vi "Create Trigger Model On Event Branch.vi"(0 "VISA resource name":refnum<visa-resource-name>, 5 "Block Number (1)":i32=1 min=1 format="%#.6g", 7 "Stimulus Event":u16(ring) items=["None", "Front Pannel Trigger Key", "Notify Trigger Block 1", "Notify Trigger Block 2", "Notify Trigger Block 3", "Notify Trigger Block 4", "Notify Trigger Block 5", "Notify Trigger Block 6", "Notify Trigger Block 7", "Notify Trigger Block 8", "Command", "Digi IO Line 1", "Digi IO Line 2", "Digi IO Line 3", "Digi IO Line 4", "Digi IO Line 5", "Digi IO Line 6", "TSP-Link 1", "TSP-Link 2", "TSP-Link 3", "LAN 1", "LAN 2", "LAN 3", "LAN 4", "LAN 5", "LAN 6", "LAN 7", "LAN 8", "Blender 1", "Blender 2", "Timer 1", "Timer 2", "Timer 3", "Timer 4", "Analog Trigger", "External Trigger"], 9 "Branch To Block":i32=1 min=1 format="%#.6g", 11 "error in (no error)":errorcluster) -> (4 "VISA resource name out":refnum<visa-resource-name>, 15 "error Out (no error)":errorcluster)   [LabVIEW 2021, in "Keithley DMM7510.lvlib"]
doc: "This VI branches to a specified block when a specified trigger event occurs."
uses:
  Keithley DMM7510.lvlib
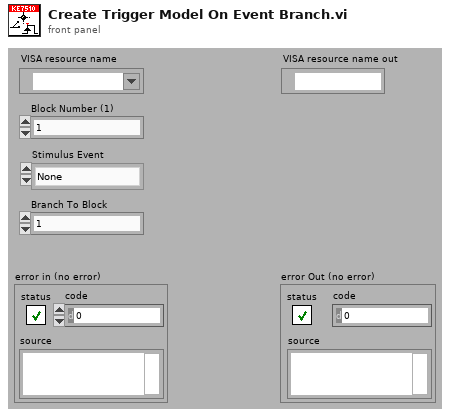
[diagram p1: front panel]
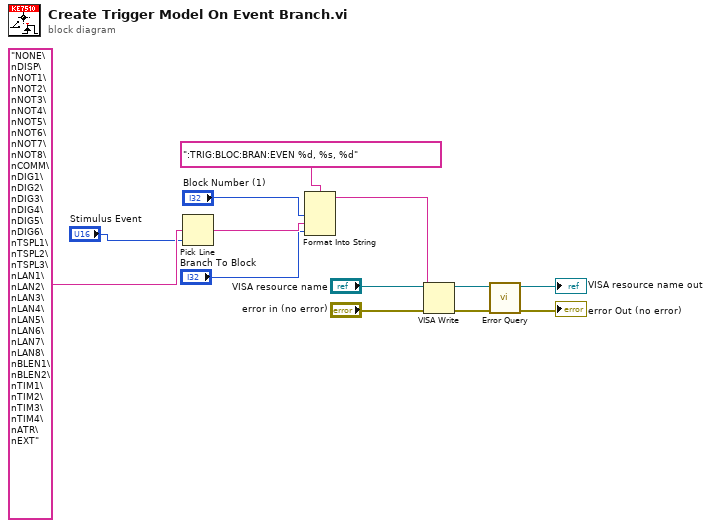
[diagram p0: block diagram]
diagram:
  n1 = Pick Line(multi-line string="NONE\nDISP\nNOT1\nNOT2\nNOT3\nNOT4\nNOT5\nNOT6\nNOT7\nNOT8\nCOMM\nDIG1\nDIG2\nDIG3\nDIG4\nDIG5\nDIG6\nTSPL1\nTSPL2\nTSPL3\nLAN1\nLAN2\nLAN3\nLAN4\nLAN5\nLAN6\nLAN7\nLAN8\nBLEN1\nBLEN2\nTIM1\nTIM2\nTIM3\nTIM4\nATR\nEXT", line index="Stimulus Event") -> (output string=w5:string)  [unwired: 1 in]
  n2 = Format Into String(format string=":TRIG:BLOC:BRAN:EVEN %d, %s, %d", "Block Number (1)", w5, "Branch To Block") -> (resulting string=w11:string)  [unwired: 2 in, 1 out]
  n3 = VISA Write(VISA resource name="VISA resource name", write buffer=w11, error in (no error)="error in (no error)") -> (VISA resource name out=w10:refnum<visa-resource-name>, error out=w9:errorcluster)  [unwired: 1 out]
  n4 = call "Error Query.vi"("error in (no error)"=w9, "VISA resource name"=w10) -> ("error out"=→"error Out (no error)":errorcluster, "VISA resource name out"=→"VISA resource name out":refnum<visa-resource-name>)  [unwired: 6 in, 2 out]
